vi "Write formula.vi"(8 "error in (no error)":errorcluster, 10 "formula":string, 11 "P in":refnum<class "P.lvclass">) -> (0 "error out":errorcluster, 3 "P out":refnum<class "P.lvclass">)   [LabVIEW 2019, in "P.lvclass"]
uses:
  P.lvclass
  P.lvclass/P.ctl
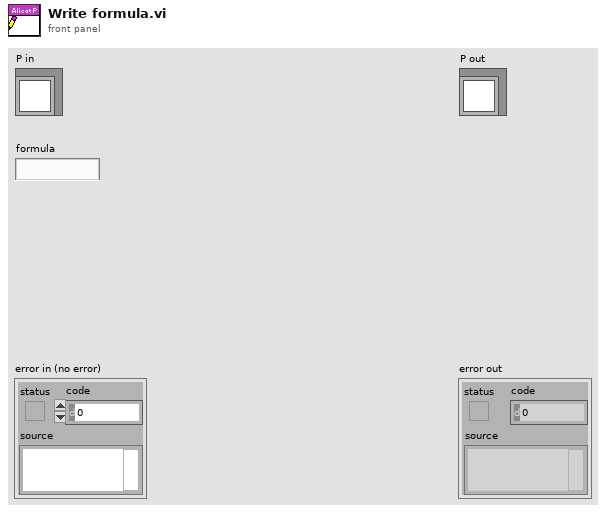
[diagram p1: front panel]
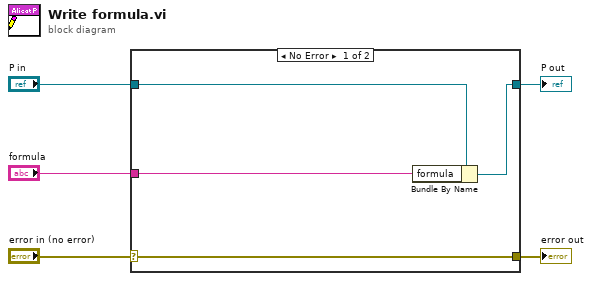
[diagram p0: block diagram]
diagram:
  n1 = case shown="No Error" "error in (no error)" {
    selector: "error in (no error)" -> [w9 w10]
    tunnel: [w9 w10] -> w4
    tunnel: [w7 w11] -> w2
    tunnel: "P in" -> [w8 w11]
    tunnel: "formula" -> [w6 _]
    frame No Error {
      n2 = Bundle By Name(cluster=w8, "formula"=w6) -> (w7:refnum<class "P.lvclass">)
    }
    frame Error {
    }
  }
  "error out" <- w4
  "P out" <- w2
